vi "instr.DSO_D.vi"(8 "错误输入（无错误）":errorcluster, 10 "CMD write":string, 11 "VISA.in":refnum<visa-resource-name>) -> (0 "错误输出":errorcluster, 1 "Reply info":string, 2 "Value":dbl, 3 "VISA.out":refnum<visa-resource-name>)   [LabVIEW 2012, in "Lib_UEL.ATE.lvlib" / "Lib_Instrument.lvlib"]
uses:
  Lib_Instrument.lvlib
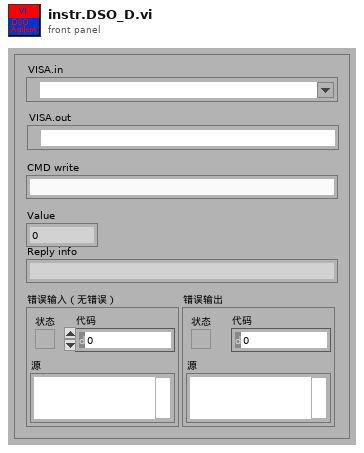
[diagram p1: front panel]
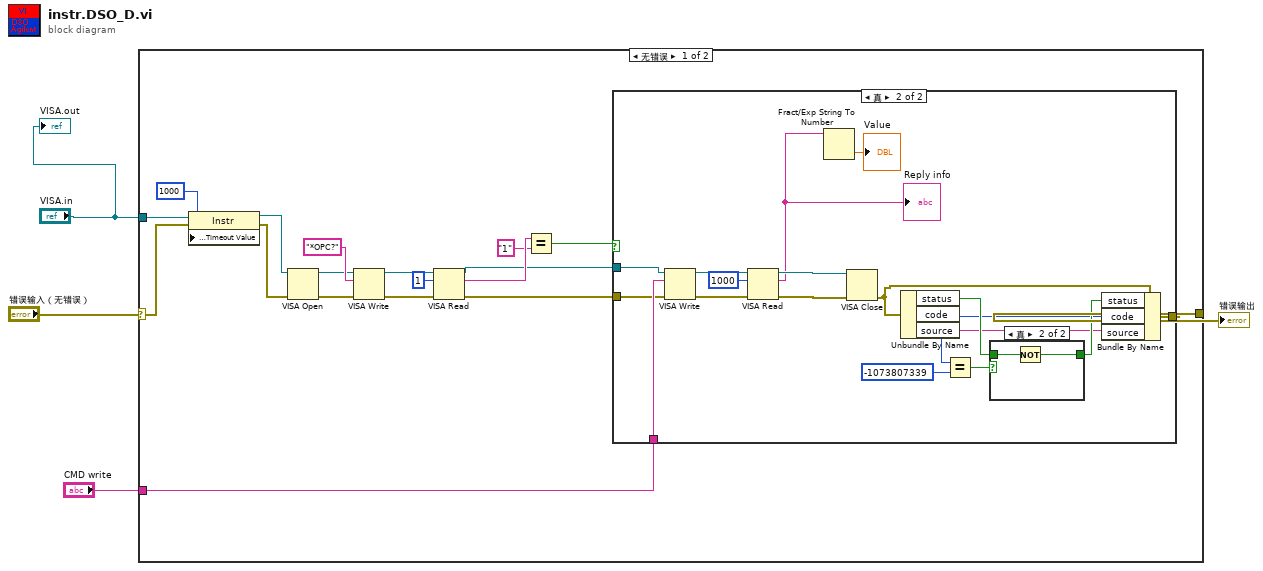
[diagram p0: block diagram]
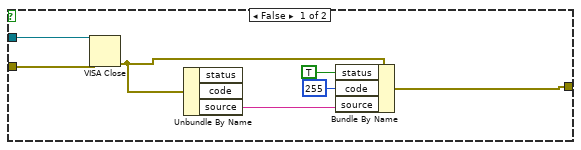
[diagram p2: hidden frame]
diagram:
  n1 = case shown="无错误" "错误输入（无错误）" {
    selector: "错误输入（无错误）" -> [w6 w51]
    tunnel: "CMD write" -> [w22 _]
    tunnel: "VISA.in" -> [w8 _]
    tunnel: [w21 w51] -> w3
    frame No Error {
      n2 = property class="Instr"(reference=w8, error in=w6, "General Settings:Timeout Value"=u32 1000) -> (reference out=w7:refnum<visa-resource-name>, error out=w5:errorcluster)
      n3 = VISA Open(error in (no error)=w5, VISA resource name=w7) -> (VISA resource name=w9:refnum<visa-resource-name>, error out=w20:errorcluster)  [unwired: 3 in]
      n4 = VISA Write(VISA resource name=w9, write buffer="*OPC?" ("写入缓冲区"), error in (no error)=w20) -> (VISA resource name out=w19:refnum<visa-resource-name>, error out=w18:errorcluster)  [unwired: 1 out]
      n5 = VISA Read(VISA resource name=w19, byte count=u32 1 ("字节总数"), error in (no error)=w18) -> (VISA resource name out=w13:refnum<visa-resource-name>, read buffer=w15:string, error out=w12:errorcluster)  [unwired: 1 out]
      n6 = Equal?(x=w15, y="1") -> (x = y?=w11:bool)
      n7 = case shown="真" w11 {
        tunnel: w22 -> [_ w43]
        tunnel: [w23 w32] -> w21
        tunnel: w13 -> [w29 w31]
        tunnel: w12 -> [w28 w30]
        frame False {
          n8 = VISA Close(VISA resource name=w29, error in (no error)=w28) -> (error out=w27:errorcluster)
          n9 = Unbundle By Name(w27) -> ("source"=w24:string)  [unwired: 2 out]
          n10 = Bundle By Name(cluster=w27, "status"=TRUE, "code"=255, "source"=w24) -> (w23:errorcluster)
        }
        frame True {
          n11 = VISA Write(VISA resource name=w31, write buffer=w43, error in (no error)=w30) -> (VISA resource name out=w44:refnum<visa-resource-name>, error out=w45:errorcluster)  [unwired: 1 out]
          n12 = VISA Read(VISA resource name=w44, byte count=u32 1000 ("字节总数"), error in (no error)=w45) -> (VISA resource name out=w46:refnum<visa-resource-name>, read buffer=w41:string, error out=w47:errorcluster)  [unwired: 1 out]
          "Reply info" <- w41
          n13 = Fract/Exp String To Number(string=w41) -> (number=→"Value":dbl)  [unwired: 3 in, 1 out]
          n14 = VISA Close(VISA resource name=w46, error in (no error)=w47) -> (error out=w36:errorcluster)
          n15 = Unbundle By Name(w36) -> ("status"=w37:bool, "code"=w34:i32, "source"=w33:string)
          n16 = Equal?(x=w34, y=-1073807339) -> (x = y?=w38:bool)
          n17 = case shown="真" w38 {
            tunnel: w37 -> [w48 w50]
            tunnel: [w48 w49] -> w35
            frame False {
            }
            frame True {
              n18 = Not(x=w50) -> (.not. x?=w49:bool)
            }
          }
          n19 = Bundle By Name(cluster=w36, "status"=w35, "code"=w34, "source"=w33) -> (w32:errorcluster)
        }
      }
    }
    frame Error {
    }
  }
  "错误输出" <- w3
  "VISA.out" <- "VISA.in"
